vi "save_collection.vi"() -> ()   [LabVIEW 2016]
uses:
  <vilib>/Utility/file.llb/Write Delimited Spreadsheet (DBL).vi
panel:
  out "Array 2":dbl[][](array[numeric])
  out "Array":dbl[][](array[numeric])
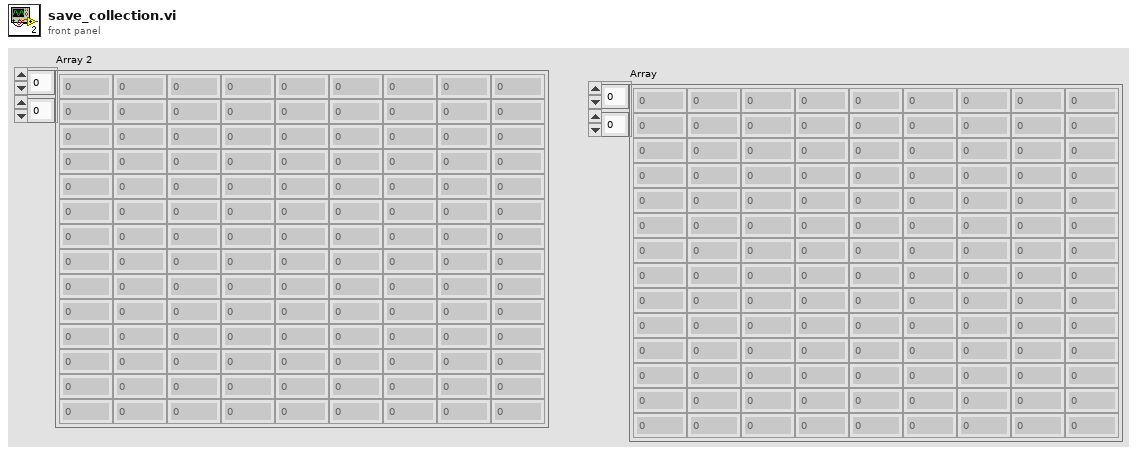
[diagram p1: front panel]
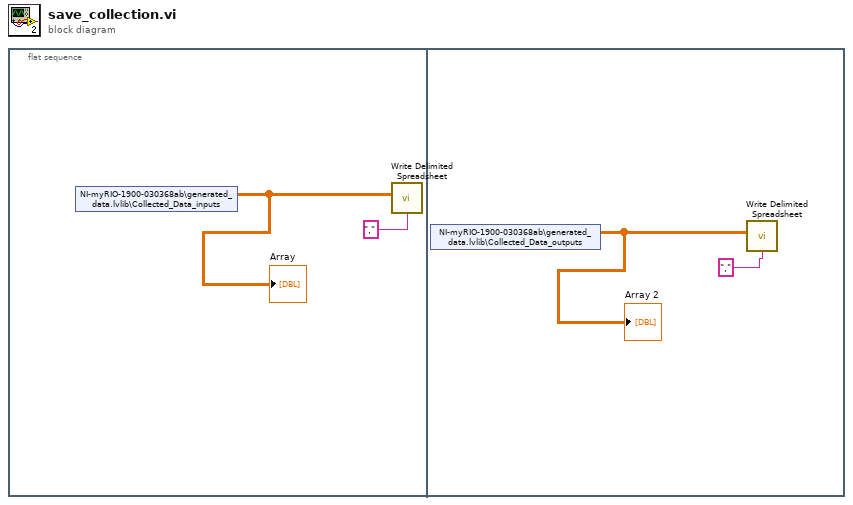
[diagram p0: block diagram]
diagram:
  n1 = flat-sequence {
    frame #0 {
      n2 = shared-variable "NI-myRIO-1900-030368ab\\generated_data.lvlib\\Collected_Data_inputs"() -> (w2:dbl[][])  [unwired: 1 in, 1 out]
      "Array" <- w2
      n3 = call-poly <vilib>:"Write Delimited Spreadsheet.vi"("2D data"=w2, "delimiter (\\t)"=",") -> ()  [unwired: 12 in, 2 out]
    }
    frame #1 {
      n4 = shared-variable "NI-myRIO-1900-030368ab\\generated_data.lvlib\\Collected_Data_outputs"() -> (w4:dbl[][])  [unwired: 1 in, 1 out]
      "Array 2" <- w4
      n5 = call-poly <vilib>:"Write Delimited Spreadsheet.vi"("2D data"=w4, "delimiter (\\t)"=",") -> ()  [unwired: 12 in, 2 out]
    }
  }
